vi "visuallyInspectPositionListResults.vi"() -> ()   [LabVIEW 2016]
uses:
  <vilib>/Utility/file.llb/Write Delimited Spreadsheet (DBL).vi
  <vilib>/regexp/Match Regular Expression.xnode
  <vilib>/vision/driver/NI_Vision_Acquisition_Software.lvlib
  <vilib>/vision/NI_Vision_Development_Module.lvlib
panel:
  out "element":i32
  in  "Camera gain":dbl(slide)=16.22568093385214 scale=0.0..20.0
  in  "Nloops":i32=1
  in  "Corner A Location [mm]":cluster{" X":dbl, "Y":dbl, "Z":dbl}={" X"=-53.53, "Y"=-29.950000000000003, "Z"=0.0}
  in  "Home?":bool
  in  "OK Button - Dump":bool
  in  "Path to save collected images":path=path "E:/BNL/XYZstage+Camera_CollectedImages/03-03-2017/images"
  in  "Process list?":T1(ring)
  in  "OK Button - Save":bool
  out "Finished!":bool
  out "Image #":i32=1
  out "Error report":errorcluster
  out "Most recently collected image":T2(plugin-control)
  out "XYZ Stage Current Position":T3={"X [-750, 750 mm]"=-652.653879887829, "Y [-150, 30 mm]"=-37.021451064321916, "Z [-50, 50 mm]"=-7.4300403600000005}
  in  "Axes Speeds [mm/s]":T4={"X Speed"=25.0, "Y Speed"=10.0, "Z Speed"=10.0}
  out "Moving":bool=TRUE
  in  "Camera Name":refnum<k21>="cam0" caption="IMAQdx Session"
  in  "Object Location [mm]":T5={"Go to X"=-451.633, "Go to Y"=-37.0215, "Go to Z"=-7.43}
  in  "error in (no error)":errorcluster
  in  "Set of Coordinates to Process":dbl[][](array[numeric])=[[-652.654, -37.0215, -7.43], [-451.633, -37.0215, -7.43], [-255.633, -37.0215, -7.43], [-59.633, -37.0215, -7.43], [136.367, -37.0215, -7.43], [332.367, -37.0215, -7.43], [528.367, -37.0215, -7.43], [528.374, -143.153, -7.43], [332.374, -143.153, -7.43], [136.374, -143.153, -7.43], [-59.626, -143.153, -7.43], [-255.626, -143.153, -7.43], [-451.626, -143.153, -7.43], [-652.654, -143.153, -7.43]]
  in  "File delimiter":string=","
  in  "List of Interesting Locations":path=path "E:/BNL/XYZstage+Camera_CollectedImages/03-03-2017/BrendonsFidMarks_dots_2017-03-03.csv"
  out "Image Array":T2[](array[plugin-control])=["image_0", "image_1", "image_2", "image_3", "image_4", "image_5", "image_6", "image_7", "image_8", "image_9", "image_10", "image_11", "image_12", "image_13", "image_14", "image_15", "image_16", "image_17", "image_18", "image_19", "image_20", "image_21", "image_22", "image_23", "image_24", "image_25", "image_26", "image_27", "image_28", "image_29", "image_30", "image_31", "image_32", "image_33", "image_34", "image_35", "image_36", "image_37", "image_38", "image_39", "image_40", "image_41", "image_42", "image_43", "image_44", "image_45", "image_46", "image_47", "image_48", "image_49", "image_50", "image_51", "image_52", "image_53", "image_54", "image_55", "image_56", "image_57", "image_58", "image_59", "image_60", "image_61", "image_62", "image_63", "image_64", "image_65", "image_66", "image_67", "image_68", "image_69", "image_70", "image_71", "image_72", "image_73", "image_74", "image_75", "image_76", "image_77", "image_78", "image_79"]
  # "Use the index box to specify the image you wish to view"
  # ">>>>"
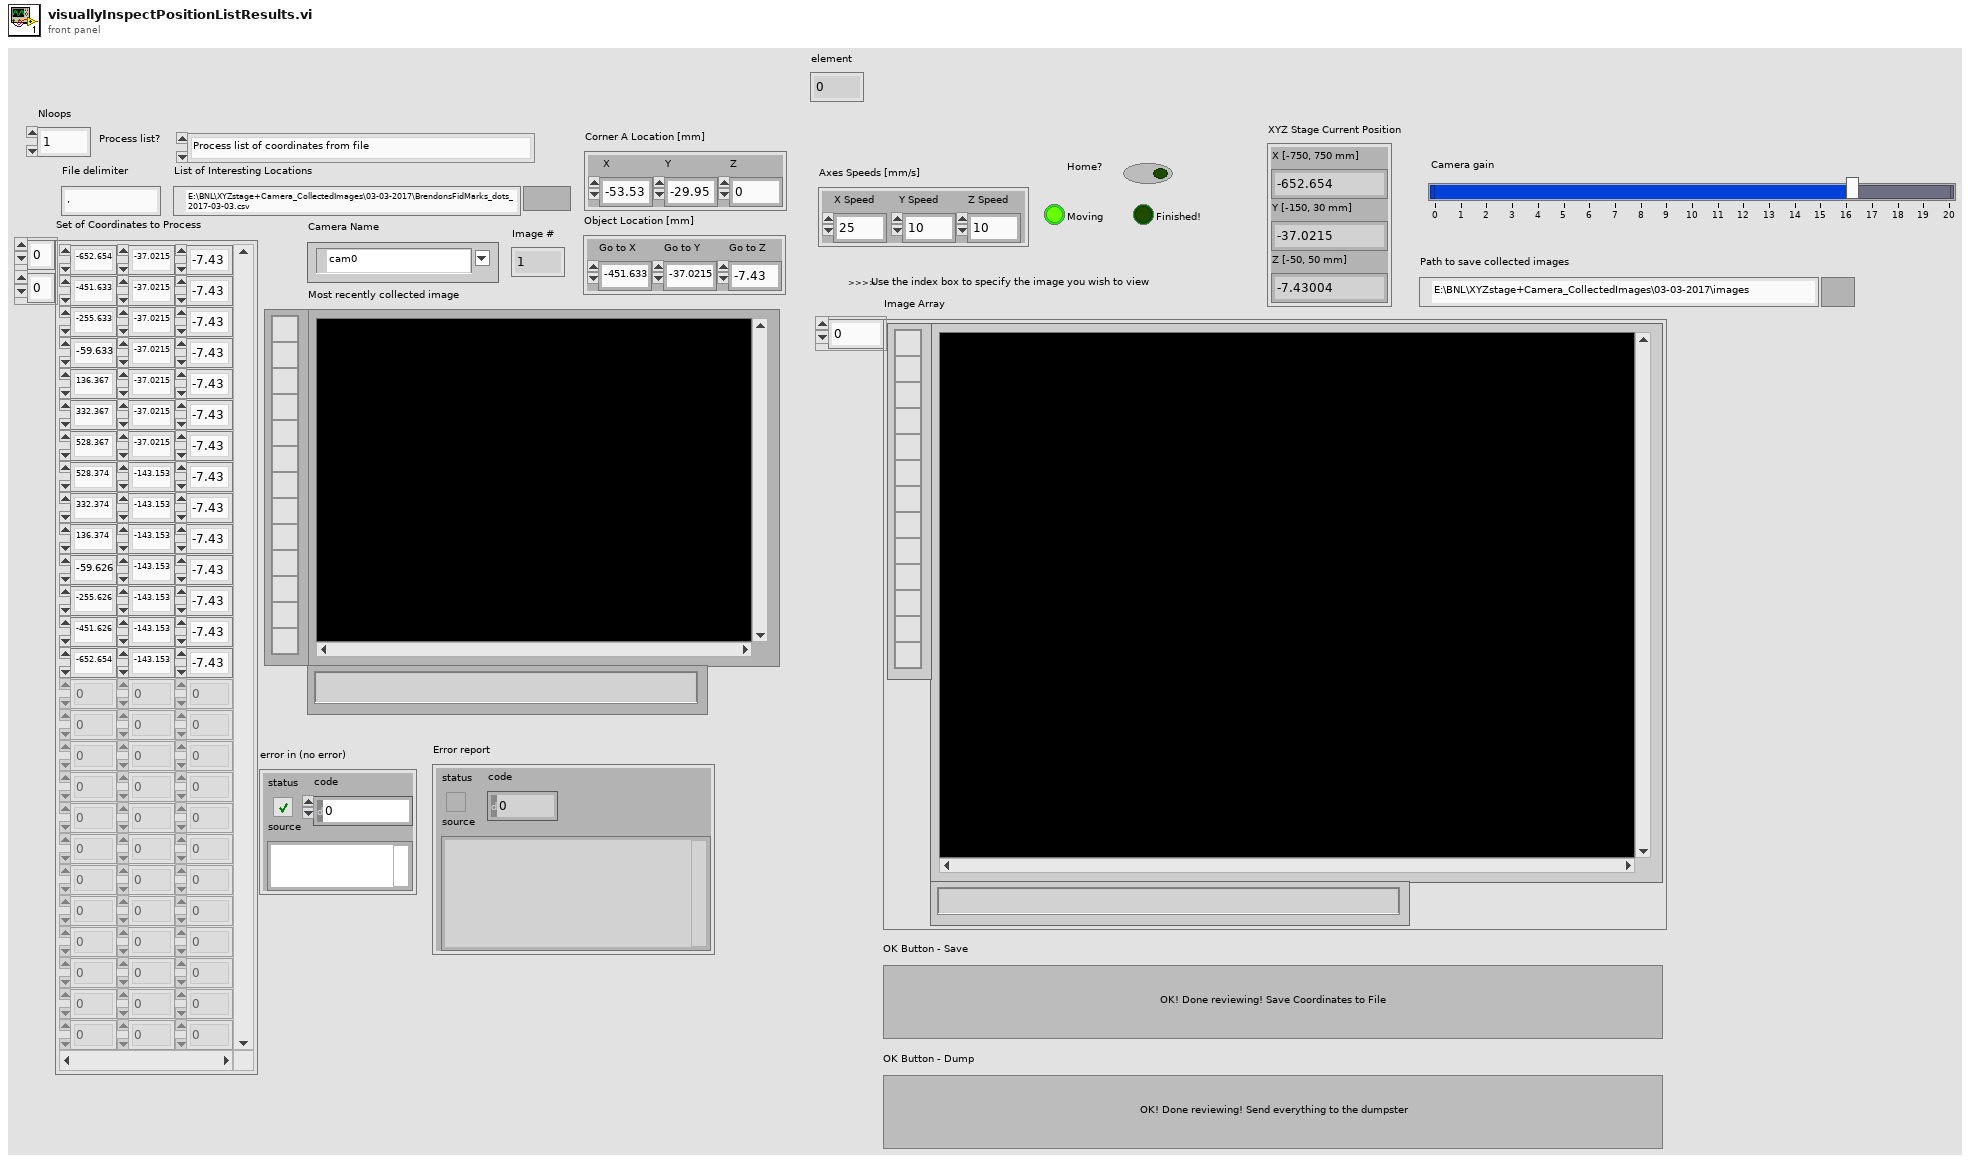
[diagram p1: front panel]
types:
  T1 = enum16{"Process list of coordinates from file", "Process list of coordinates entered manually", "Generate list based on initial coordinate"}
  T2 = typedef "IMAQ Image.ctl" = refnum<image>
  T3 = cluster{"X [-750, 750 mm]":dbl, "Y [-150, 30 mm]":dbl, "Z [-50, 50 mm]":dbl}
  T4 = cluster{"X Speed":dbl, "Y Speed":dbl, "Z Speed":dbl}
  T5 = cluster{"Go to X":dbl, "Go to Y":dbl, "Go to Z":dbl}
  T6 = typedef "IMAQdx.ctl" = refnum<k21>
  T7 = cluster{"Set of Coordinates to Process[0]":dbl, "Set of Coordinates to Process[1]":dbl, "Set of Coordinates to Process[2]":dbl}
  T8 = typedef "Image Type" = u32
  T9 = cluster{"Final X":dbl, "Final Y":dbl, "Final Z":dbl}
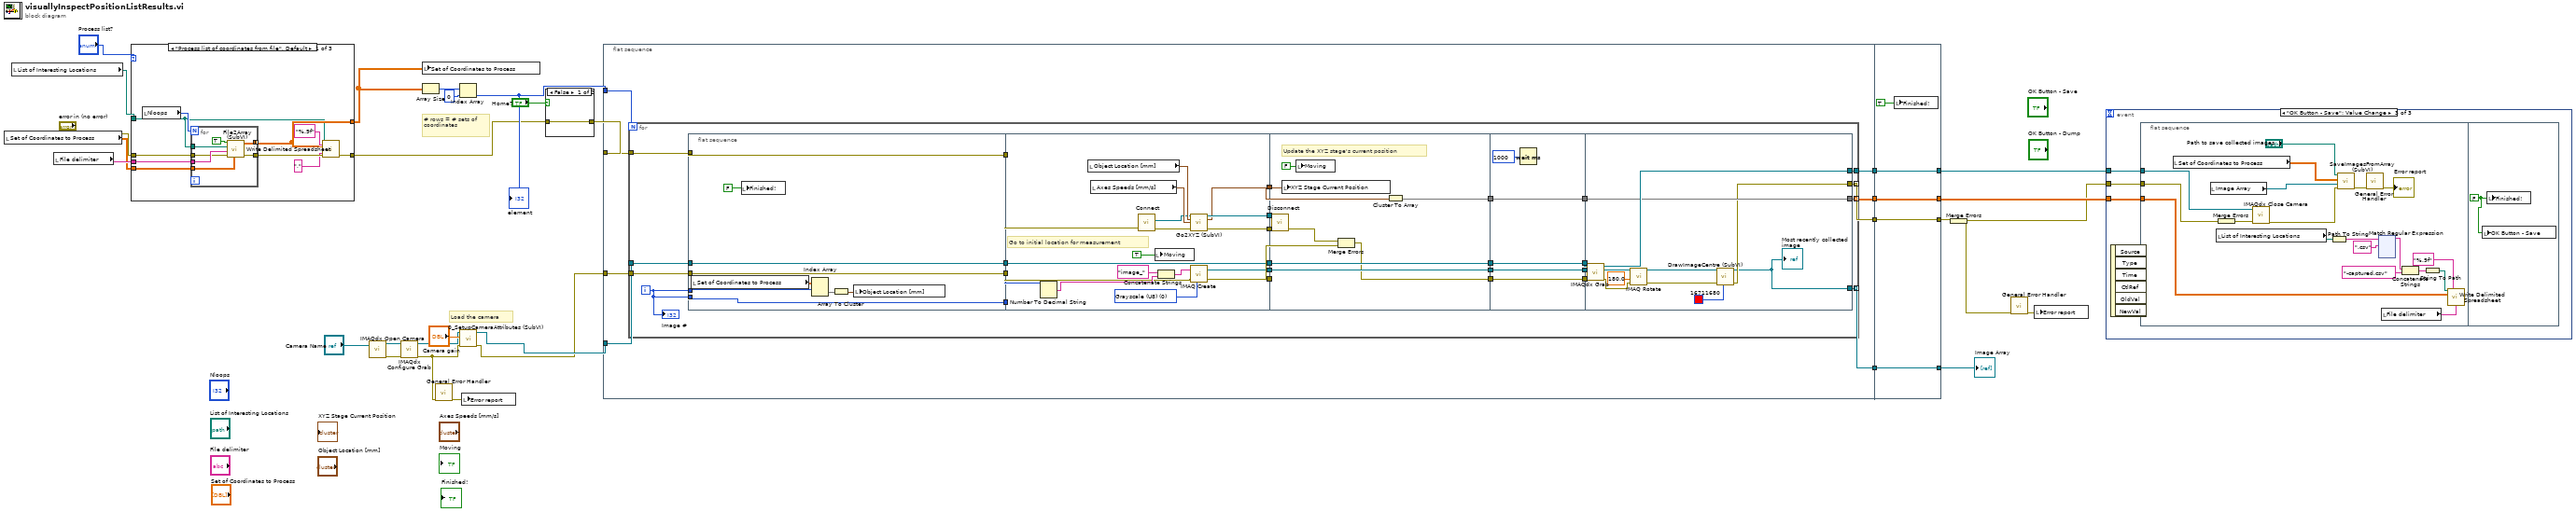
[diagram p0: block diagram]
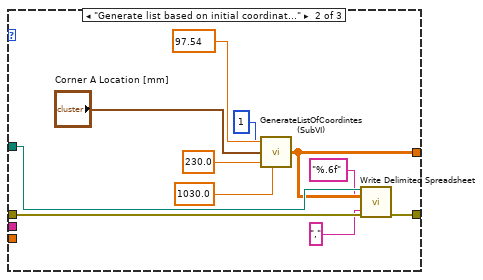
[diagram p2: hidden frame]
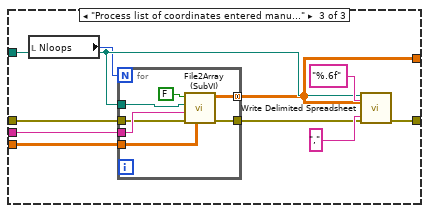
[diagram p3: hidden frame]
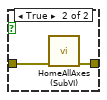
[diagram p4: hidden frame]
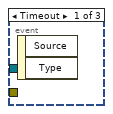
[diagram p5: hidden frame]
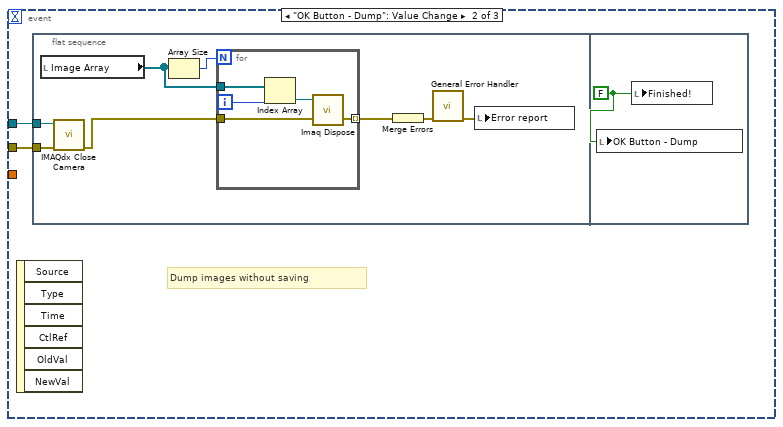
[diagram p6: hidden frame]
diagram:
  # "# rows = # sets of\ncoordinates"
  # "Load the camera"
  n1 = local read "Set of Coordinates to Process"() -> (w11:dbl[][])
  n2 = local read "List of Interesting Locations"() -> (w10:path)
  n3 = local read "File delimiter"() -> (w13:string)
  n4 = case shown="\"Process list of coordinates from file\", Default" "Process list?" {
    tunnel: [w35 w52 w61] -> w22
    tunnel: [w34 w54 w63] -> w15
    tunnel: w13 -> [w41 _ w69]
    tunnel: "error in (no error)" -> [w40 w53 w68]
    tunnel: w11 -> [w39 _ w67]
    tunnel: w10 -> [w33 w55 w64]
    frame "Process list of coordinates from file", Default {
      n5 = local read "Nloops"() -> (w38:i32)
      n6 = for {
        N: w38 -> [_]
        tunnel: w33 -> [w45]
        tunnel: w41 -> [w44]
        tunnel: w39 -> [w42]
        tunnel: [w48] -> w34 mode=concatenating
        tunnel: w40 -> [w43]
        tunnel: [w47] -> w36
        n7 = call "File2Array (SubVI).vi"("Array for Processing"=w42, "error in (no error) in"=w43, "File delimiter"=w44, "Source array file"=w45, "Load array from file?"=TRUE) -> ("error in (no error) out"=w47:errorcluster, "Loaded array"=w48:dbl[][])  [unwired: 5 in]
      }
      n8 = call-poly <vilib>:"Write Delimited Spreadsheet.vi"("file path (dialog if empty)"=w33, "format (%.3f)"="%.9f", "2D data"=w34, "error in (no error)"=w36, "delimiter (\\t)"="," ("delimiter (\\t)")) -> ("error out"=w35:errorcluster)  [unwired: 9 in, 1 out]
    }
    frame "Generate list based on initial coordinate" {
      n9 = call "GenerateListOfCoordintes (SubVI).vi"("Module side length [mm]"=97.54, "Nloops"=1, "A [mm]"="Corner A Location [mm]", "x to fiducial [um]"=230.0, "y to fiducial [um]"=1030.0) -> ("Generated List of Coordinates"=w54:dbl[][])  [unwired: 4 in]
      n10 = call-poly <vilib>:"Write Delimited Spreadsheet.vi"("file path (dialog if empty)"=w55, "format (%.3f)"="%.6f", "2D data"=w54, "error in (no error)"=w53, "delimiter (\\t)"="," ("delimiter (\\t)")) -> ("error out"=w52:errorcluster)  [unwired: 9 in, 1 out]
    }
    frame "Process list of coordinates entered manually" {
      n11 = local read "Nloops"() -> (w60:i32)
      n12 = for {
        N: w60 -> [_]
        tunnel: w69 -> [w75]
        tunnel: w64 -> [w72]
        tunnel: w67 -> [w73]
        tunnel: [w71] -> w63 mode=concatenating
        tunnel: w68 -> [w74]
        tunnel: [w70] -> w62
        n13 = call "File2Array (SubVI).vi"("Array for Processing"=w73, "error in (no error) in"=w74, "File delimiter"=w75, "Source array file"=w72, "Load array from file?"=FALSE) -> ("error in (no error) out"=w70:errorcluster, "Loaded array"=w71:dbl[][])  [unwired: 5 in]
      }
      n14 = call-poly <vilib>:"Write Delimited Spreadsheet.vi"("file path (dialog if empty)"=w64, "format (%.3f)"="%.6f", "2D data"=w63, "error in (no error)"=w62, "delimiter (\\t)"="," ("delimiter (\\t)")) -> ("error out"=w61:errorcluster)  [unwired: 9 in, 1 out]
    }
  }
  n15 = call <vilib>:"IMAQdx Open Camera.vi"("Session In"="Camera Name") -> ("error out"=w27:errorcluster, "Session Out"=w28:T6)  [unwired: 2 in, 7 out]
  n16 = call <vilib>:"IMAQdx Configure Grab.vi"("error in"=w27, "Session In"=w28) -> ("error out"=w4:errorcluster, "Session Out"=w3:T6)  [unwired: 8 out]
  n17 = local write "Set of Coordinates to Process"(w15) -> ()
  n18 = Array Size(array=w15) -> (size(s)=w31:i32[])
  n19 = call <vilib>:"General Error Handler.vi"("error in (no error)"=w4) -> ("error out"=w17:errorcluster)  [unwired: 2 in, 12 out]
  n20 = Index Array(array=w31, index=0) -> (element=w29:i32)
  "element" <- w29
  n21 = call "0_SetupCameraAttributes (SubVI).vi"("error in (no error)"=w4, "Gain"="Camera gain", "Camera session in"=w3) -> ("error out"=w1:errorcluster, "Camera session out"=w2:T6)  [unwired: 7 in]
  n22 = local write "Error report"(w17) -> ()
  n23 = case shown="False" "Home?" {
    tunnel: w22 -> [w77 w79]
    tunnel: [w77 w78] -> w21
    frame False {
    }
    frame True {
      n24 = call "HomeAllAxes (SubVI).vi"("error in (no error)"=w79) -> ("error out"=w78:errorcluster)  [unwired: 8 in, 2 out]
    }
  }
  n25 = flat-sequence {
    tunnel: w29 -> [w87]
    tunnel: w2 -> [w86]
    tunnel: w21 -> [w82]
    tunnel: w1 -> [w80]
    tunnel: [w85] -> w9
    tunnel: [w84] -> w8
    tunnel: [w83] -> w7
    tunnel: [w81] -> w6
    tunnel: [w170] -> w20
    tunnel: [w171] -> w23
    tunnel: [w172] -> w24
    tunnel: [w173] -> w25
    tunnel: w9 -> [w173]
    tunnel: w8 -> [w172]
    tunnel: w7 -> [w171]
    tunnel: w6 -> [w170]
    frame #0 {
      n26 = for {
        N: w87 -> [_]
        tunnel: w86 -> [w101]
        tunnel: [w100] -> w85 mode=indexing
        tunnel: w82 -> [w98]
        tunnel: w80 -> [w96]
        tunnel: [w92] -> w84
        tunnel: [w91] -> w81 mode=indexing
        tunnel: [w88] -> w83 mode=indexing
        i -> [w109]
        n27 = flat-sequence {
          tunnel: w109 -> [w119]
          tunnel: w109 -> [w118]
          tunnel: [w118] -> w110
          tunnel: [w117] -> w102
          tunnel: w101 -> [w117]
          tunnel: [w116] -> w99
          tunnel: w98 -> [w116]
          tunnel: [w115] -> w97
          tunnel: w96 -> [w115]
          tunnel: [w134] -> w113
          tunnel: [w133] -> w112
          tunnel: [w132] -> w111
          tunnel: w110 -> [w127]
          tunnel: [w129] -> w106
          tunnel: [w128] -> w103
          tunnel: w102 -> [w128]
          tunnel: w99 -> [w125]
          tunnel: w97 -> [w124]
          tunnel: [w123] -> w93
          tunnel: w113 -> [w149]
          tunnel: w112 -> [w142]
          tunnel: w111 -> [w148]
          tunnel: [w147] -> w107
          tunnel: w106 -> [w147]
          tunnel: [w146] -> w104
          tunnel: w103 -> [w146]
          tunnel: [w143] -> w94
          tunnel: w93 -> [w144]
          tunnel: [w141] -> w90
          tunnel: [w154] -> w108
          tunnel: w107 -> [w154]
          tunnel: [w153] -> w105
          tunnel: w104 -> [w153]
          tunnel: [w152] -> w95
          tunnel: w94 -> [w152]
          tunnel: w90 -> [w151]
          tunnel: [w151] -> w89
          tunnel: w108 -> [w168]
          tunnel: w105 -> [w167]
          tunnel: [w157] -> w100
          tunnel: w95 -> [w164]
          tunnel: [w162] -> w92
          tunnel: [w158] -> w91
          tunnel: w89 -> [w161]
          tunnel: [w161] -> w88
          frame #0 {
            n28 = local read "Set of Coordinates to Process"() -> (w120:dbl[][])
            n29 = local write "Finished!"(FALSE ("Finished!")) -> ()
            n30 = Index Array(array=w120, index (row)=w119) -> (element=w121:dbl[])  [unwired: 1 in]
            n31 = Array To Cluster(array=w121) -> (cluster=w122:T7)
            n32 = local write "Object Location [mm]"(w122) -> ()
          }
          frame #1 {
            w140 = T8 0 items=["Grayscale (U8)", "Grayscale (I16)", "Grayscale (SGL)", "Complex (CSG)", "RGB (U32)", "HSL (U32)", "RGB (U64)", "Grayscale (U16)"] ("Image Type")
            # "Go to initial location for measurement"
            n33 = Number To Decimal String(number=w127) -> (decimal integer string=w126:string)  [unwired: 1 in]
            n34 = local read "Object Location [mm]"() -> (w137:T5)
            n35 = local read "Axes Speeds [mm/s]"() -> (w138:T4)
            n36 = call "Connect.vi"("error in (no error)"=w125) -> ("error out"=w135:errorcluster, "controller"=w136:refnum<k24>)  [unwired: 9 in]
            n37 = local write "Moving"(TRUE ("Moving")) -> ()
            n38 = Concatenate Strings("image_" ("Image Name"), w126) -> (w130:string)
            n39 = call "Go2XYZ (SubVI).vi"(".NET Refnum in"=w136, "Go to Coordinates"=w137, "Axis Speeds"=w138, "error in (no error)"=w135) -> (".NET Refnum out"=w134:refnum<k24>, "Final Position"=w133:T9, "error out"=w132:errorcluster)  [unwired: 8 in, 1 out]
            n40 = call "IMAQ Create"("Image Name"=w130, "Image Type"=w140, "error in (no error)"=w124) -> ("New Image"=w129:T2, "error out"=w123:errorcluster)  [unwired: 1 in, 1 out]
          }
          frame #2 {
            # "Update the XYZ stage's current position"
            n41 = call "Disconnect.vi"("error in (no error)"=w148, "controller"=w149) -> ("error out"=w145:errorcluster)  [unwired: 9 in]
            n42 = local write "XYZ Stage Current Position"(w142) -> ()
            n43 = local write "Moving"(FALSE ("Moving")) -> ()
            n44 = Merge Errors(w145, w144) -> (w143:errorcluster)
            n45 = Cluster To Array(cluster=w142) -> (array=w141:dbl[])
          }
          frame #3 {
            n46 = Wait (ms)(milliseconds to wait=u32 1000) -> ()  [unwired: 1 out]
          }
          frame #4 {
            n47 = call <vilib>:"IMAQdx Grab.vi"("error in"=w164, "Image In"=w168, "Session In"=w167) -> ("error out"=w163:errorcluster, "Image Out"=w166:T2, "Session Out"=w162:T6)  [unwired: 1 in, 5 out]
            n48 = call "IMAQ Rotate"("error in (no error)"=w163, "Angle (degrees)"=sgl 180.0, "Image Src"=w166) -> ("error out"=w159:errorcluster, "Image Dst Out"=w160:T2)  [unwired: 7 in]
            n49 = call "DrawImageCentre (SubVI).vi"("Axis colour"=u32 16711680, "error in (no error)"=w159, "Refnum in"=w160) -> ("error out"=w158:errorcluster, "Refnum out"=w157:T2)  [unwired: 7 in]
            "Most recently collected image" <- w157
          }
        }
        "Image #" <- w109
      }
    }
    frame #1 {
      n50 = local write "Finished!"(TRUE ("Finished!")) -> ()
    }
  }
  n51 = Merge Errors(w20) -> (w18:errorcluster)
  n52 = call <vilib>:"General Error Handler.vi"("error in (no error)"=w18) -> ("error out"=w19:errorcluster)  [unwired: 2 in, 12 out]
  n53 = local write "Error report"(w19) -> ()
  n54 = event shown="[2] \"OK Button - Save\": Value Change" {
    selector: _ -> [_ _ _]
    dyn-events: _ -> [_ _ _]
    timeout: _ -> [_ _ _]
    tunnel: w18 -> [_ w174 w192]
    tunnel: w24 -> [_ w175 w191]
    tunnel: w23 -> [_ _ w190]
    event Timeout {
      n55 = event-data() -> ()  [unwired: 1 in, 2 out]
    }
    event "OK Button - Dump": Value Change {
      # "Dump images without saving"
      n56 = event-data() -> ()  [unwired: 1 in, 6 out]
      n57 = flat-sequence {
        tunnel: w175 -> [w183]
        tunnel: w174 -> [w182]
        frame #0 {
          n58 = local read "Image Array"() -> (w181:T2[])
          n59 = call <vilib>:"IMAQdx Close Camera.vi"("error in"=w182, "Session In"=w183) -> ("error out"=w178:errorcluster)  [unwired: 9 out]
          n60 = Array Size(array=w181) -> (size(s)=w180:i32)
          n61 = for {
            N: w180 -> [_]
            tunnel: w181 -> [w188]
            tunnel: w178 -> [w185]
            tunnel: [w184] -> w177 mode=indexing
            i -> [w187]
            n62 = Index Array(array=w188, index=w187) -> (element=w186:T2)
            n63 = call "Imaq Dispose"("Image"=w186, "error in (no error)"=w185) -> ("error out"=w184:errorcluster)  [unwired: 4 in]
          }
          n64 = Merge Errors(w177) -> (w176:errorcluster)
          n65 = call <vilib>:"General Error Handler.vi"("error in (no error)"=w176) -> ("error out"=w179:errorcluster)  [unwired: 2 in, 12 out]
          n66 = local write "Error report"(w179) -> ()
        }
        frame #1 {
          w189 = FALSE ("Finished!")
          n67 = local write "OK Button - Dump"(w189) -> ()
          n68 = local write "Finished!"(w189) -> ()
        }
      }
    }
    event "OK Button - Save": Value Change {
      n69 = event-data() -> ()  [unwired: 1 in, 6 out]
      n70 = flat-sequence {
        tunnel: w192 -> [w201]
        tunnel: w191 -> [w200]
        tunnel: w190 -> [w199]
        frame #0 {
          n71 = local read "Set of Coordinates to Process"() -> (w194:dbl[][])
          n72 = local read "Image Array"() -> (w198:T2[])
          n73 = local read "List of Interesting Locations"() -> (w204:path)
          n74 = Merge Errors(w201) -> (w202:errorcluster)
          n75 = call <vilib>:"IMAQdx Close Camera.vi"("error in"=w202, "Session In"=w200) -> ("error out"=w197:errorcluster)  [unwired: 9 out]
          n76 = Path To String(path=w204) -> (string=w205:string)
          n77 = call "SaveImagesFromArray (SubVI).vi"("error in (no error)"=w197, "Array of Images"=w198, "XY Camera Coordinates"=w194, "Path to save collected images"="Path to save collected images") -> ("error out"=w196:errorcluster)  [unwired: 7 in]
          n78 = call <vilib>:"General Error Handler.vi"("error in (no error)"=w196) -> ("error out"=→"Error report":errorcluster)  [unwired: 2 in, 12 out]
          n79 = xnode "Match Regular Expression"("input string"=w205, "regular expression"=".csv") -> ("before match"=w208:string)  [unwired: 4 in, 4 out]
          n80 = local read "File delimiter"() -> (w211:string)
          n81 = Concatenate Strings(w208, "-captured.csv" ("name or relative path")) -> (w209:string)
          n82 = String To Path(string=w209) -> (path=w210:path)
          n83 = call-poly <vilib>:"Write Delimited Spreadsheet.vi"("file path (dialog if empty)"=w210, "format (%.3f)"="%.9f", "2D data"=w199, "delimiter (\\t)"=w211) -> ()  [unwired: 10 in, 2 out]
        }
        frame #1 {
          w326 = FALSE ("Finished!")
          n84 = local write "OK Button - Save"(w326) -> ()
          n85 = local write "Finished!"(w326) -> ()
        }
      }
    }
  }
  "Image Array" <- w25
